vi "FPGA_AIReadLSBWeight.vi"(8 "error in (no error)":errorcluster, 10 "Channel":T1, 11 "AI Reference":T2) -> (0 "error out":errorcluster, 2 "LSBWeight":u32, 3 "AI Reference":T2)   [LabVIEW 2017]
uses:
  <vilib>/Rock Robotics/SystemInterfaces/AI/FPGA_AIDevRef.ctl
  <vilib>/Rock Robotics/SystemInterfaces/AI/FPGA_AIChannel.ctl
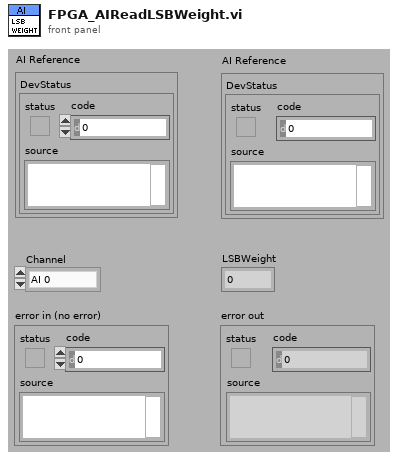
[diagram p1: front panel]
types:
  T1 = typedef "FPGA_AIChannel.ctl" = enum8{"AI 0", "AI 1", "AI 2", "AI 3", "AI MXP 0", "AI MXP 1", "AI MXP 2", "AI MXP 3", "Invalid"}
  T2 = typedef "FPGA_AIDevRef.ctl" = cluster{"DevStatus":errorcluster}
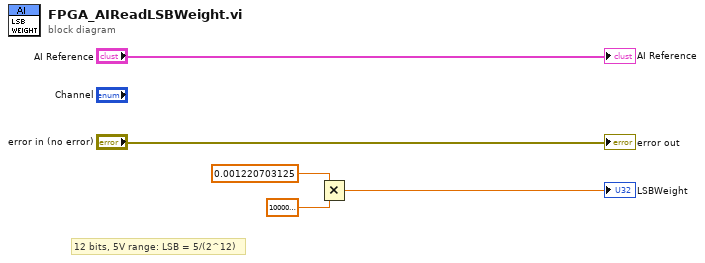
[diagram p0: block diagram]
diagram:
  # "12 bits, 5V range: LSB = 5/(2^12)"
  n1 = Multiply(x=0.001220703125 ("y"), y=1000000000.0) -> (x*y=→"LSBWeight":dbl)
  "AI Reference" <- "AI Reference"
  "error out" <- "error in (no error)"
